vi "Begin.vi"(11 "Image Size":T4=enum."160x120") -> (0 "error out":errorcluster)   [LabVIEW 2012]
doc: "Called before other user functions, this VI is expected to open initial I/O refnums, load in file data, and do all program initialization. Notice that the <B>error out</B> terminal is simply used for data flow. Wiring it to other structures or subVIs ensures that this VI runs first."
uses:
  <vilib>/Rock Robotics/WPI/Camera/WPI_CameraImageSize.ctl
  <vilib>/Rock Robotics/SystemInterfaces/DIO/FPGA_DIOChannel.ctl
  <vilib>/Rock Robotics/WPI/Encoder/WPI_EncoderType.ctl
  <vilib>/Rock Robotics/SystemInterfaces/Typedef/FPGA_TypedefDigitalModule.ctl
  <vilib>/Rock Robotics/WPI/Camera/WPI_CameraWhite Balance Values.ctl
  <vilib>/Rock Robotics/WPI/Camera/WPI_CameraExposure Values.ctl
  <vilib>/Rock Robotics/WPI/Camera/WPI_CameraFrameRate.ctl
  <vilib>/Rock Robotics/WPI/DriverStation/WPI_DriverStationRobotMode2.ctl
  <vilib>/Rock Robotics/WPI/Joystick/WPI_JoystickDeviceEnum.ctl
  <vilib>/Rock Robotics/SystemInterfaces/Typedef/FPGA_TypedefAnalogModuleForGyro.ctl
  <vilib>/Rock Robotics/SystemInterfaces/AI/FPGA_AIGyroChannel.ctl
  <vilib>/Rock Robotics/WPI/SafetyOutput/WPI_SafetyOutputConfigMenu.ctl
  <vilib>/Rock Robotics/WPI/CAN/Jaguar/SubVIs/WPI_CANJaguar_ControlMode.ctl
  Robot Global Data.vi
  <vilib>/Rock Robotics/WPI/Counter/WPI_CounterDigitalInputToDigitalSource.vi
  <vilib>/Rock Robotics/WPI/MotorControl/WPI_MotorControlOpenCANJaguar.vi
  <vilib>/Rock Robotics/WPI/RobotDrive/WPI_RobotDriveOpen4MotorWithExistingMotors.vi
panel:
  in  "DIO Module":T1
  in  "Invert Direction":bool
  in  "Decoding Type":T2=enum."4x"
  in  "DistancePerCount (deg)":dbl=0.288
  in  "Encoder B Channel":T3=enum."DIO 2"
  in  "Encoder A Channel":T3
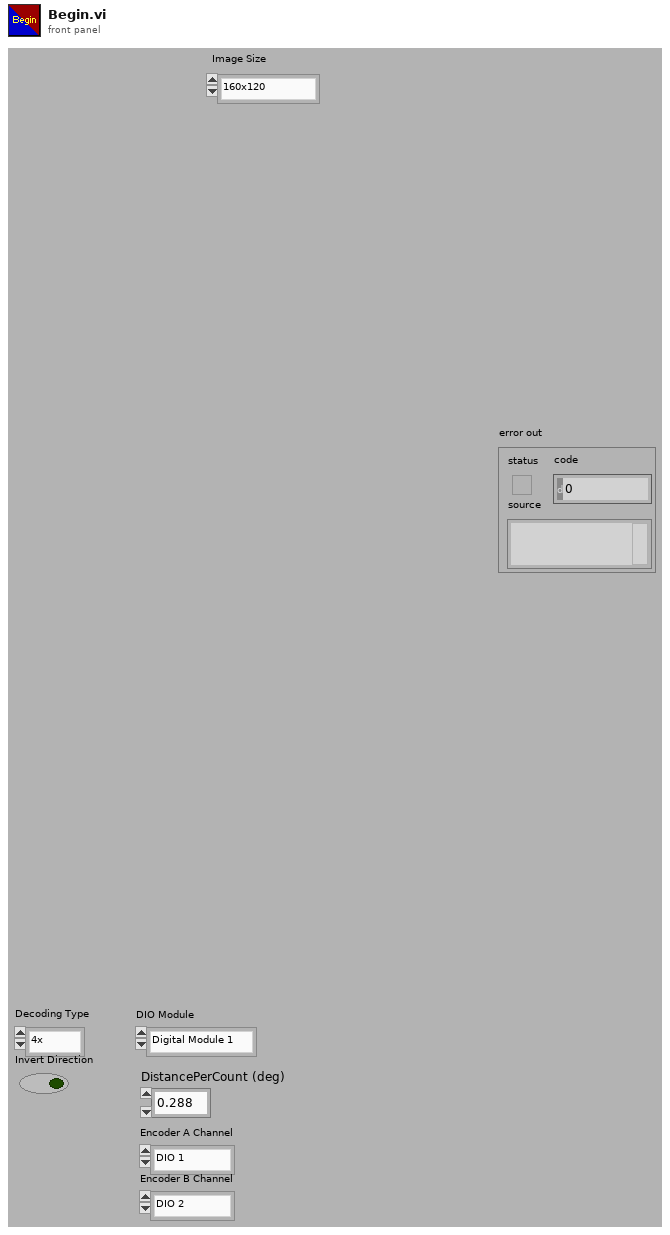
[diagram p1: front panel]
types:
  T1 = typedef "FPGA_TypedefDigitalModule.ctl" = enum16{"Digital Module 1", "Digital Module 2"}
  T2 = typedef "WPI_EncoderType.ctl" = enum16{"1x", "2x", "4x"}
  T3 = typedef "FPGA_DIOChannel.ctl" = enum8{"DIO 1", "DIO 2", "DIO 3", "DIO 4", "DIO 5", "DIO 6", "DIO 7", "DIO 8", "DIO 9", "DIO 10", "DIO 11", "DIO 12", "DIO 13", "DIO 14", "Invalid"}
  T4 = typedef "WPI_CameraImageSize.ctl" = enum16{"640x480", "320x240", "160x120"}
  T5 = typedef "WPI_CANJaguar_ControlMode.ctl" = enum8{"Percent VBus", "Current", "Speed", "Position", "Voltage"}
  T6 = typedef "WPI_SafetyOutputConfigMenu.ctl" = enum16{"Enable", "Disable"}
  T7 = typedef "FPGA_AIGyroChannel.ctl" = enum8{"AI 1", "AI 2", "Invalid"}
  T8 = typedef "FPGA_TypedefAnalogModuleForGyro.ctl" = enum16{"Analog Module 1"}
  T9 = typedef "WPI_JoystickDeviceEnum.ctl" = enum16{"USB 1", "USB 2", "USB 3", "USB 4", "Kinect 1", "Kinect 2"}
  T10 = typedef "WPI_DriverStationRobotMode2.ctl" = enum16{"Autonomous Disabled", "Autonomous Enabled", "Teleop Disabled", "Teleop Enabled", "Timeout", "Finish", "Test Disabled", "Test Enabled"}
  T11 = typedef "WPI_CameraFrameRate.ctl" = u32
  T12 = typedef "WPI_CameraExposure Values.ctl" = enum16{"Auto", "Flicker-free 50 Hz", "Flicker-free 60 Hz", "Hold current"}
  T13 = typedef "WPI_CameraWhite Balance Values.ctl" = enum16{"Auto", "Fixed indoor", "Fixed outdoor 1", "Fixed outdoor 2", "Fixed fluorescent 1", "Fixed fluorescent 2", "Hold current"}
  T14 = typedef "WPI_GyroDevRef.ctl" = cluster{"DevStatus":errorcluster, "Analog Module":T15, "Analog Channel":T16, "Offset":dbl, "Gain (VoltsPerDegree/Second)":dbl}
  T15 = typedef "FPGA_TypedefAnalogModule.ctl" = enum16{"Analog Module 1", "Analog Module 2"}
  T16 = typedef "FPGA_AIChannel.ctl" = enum8{"AI 1", "AI 2", "AI 3", "AI 4", "AI 5", "AI 6", "AI 7", "AI 8", "Invalid"}
  T17 = typedef "WPI_MotorControlDeviceRef.ctl" = cluster{"DeviceStatus":errorcluster, "Type":enum16{"PWM", "CAN"}, "PWM":cluster{"Digital Module":T1, "PWM Channel":T18, "DeadBand":T19}, "CAN":cluster{"Device Number":u8, "Control Mode":T5, "Semaphore":T20, "Max Vout":dbl}, "Invert":bool, "TransformRef":T21, "InvTransformRef":T21}
  T18 = typedef "FPGA_DIOPWMChannel.ctl" = enum8{"PWM 1", "PWM 2", "PWM 3", "PWM 4", "PWM 5", "PWM 6", "PWM 7", "PWM 8", "PWM 9", "PWM 10", "Invalid"}
  T19 = typedef "WPI_PWMDeadband.ctl" = cluster{"Name":string, "maxPositivePwm":i32, "minPositivePwm":i32, "centerPwm":i32, "maxNegativePwm":i32, "minNegativePwm":i32, "angularRange":u16}
  T20 = typedef "Semaphore RefNum" = refnum<k1>
  T21 = typedef "WPI_PWMTransform_ConPane.ctl" = refnum<vi>
  T22 = typedef "WPI_DigitalInputDevRef.ctl" = cluster{"DevStatus":errorcluster, "DIO Channel":T3, "Digital Module":T1}
  T23 = typedef "WPI_CameraDevRef.ctl" = cluster{"Camera Address":string, "CameraStatus":errorcluster, "Acquire Image Notifier":refnum<notifier>}
  T24 = typedef "WPI_JoystickDevRef.ctl" = cluster{"Device":T9}
  T25 = typedef "FPGA_CounterEncoderSourceConvertionLVSourceType.ctl" = cluster{"DevStatus":errorcluster, "AnalogTriggerMode?":bool, "DigitalMode":cluster{"Digital Module":T1, "DIO Channel":T26}, "AnalogTriggerMode":cluster{"AnalogTriggerIndex":T27, "OutputType":T28}}
  T26 = typedef "FPGA_DIODigitalSourceChannel.ctl" = enum8{"DIO 1", "DIO 2", "DIO 3", "DIO 4", "DIO 5", "DIO 6", "DIO 7", "DIO 8", "DIO 9", "DIO 10", "DIO 11", "DIO 12", "DIO 13", "DIO 14", "Disabled"}
  T27 = typedef "FPGA_AnalogTriggerIndex.ctl" = enum8{"Trig 0", "Trig 1", "Trig 2", "Trig 3", "Trig 4", "Trig 5", "Trig 6", "Trig 7", "Invalid"}
  T28 = typedef "FPGA_AnalogTriggerOutType.ctl" = enum16{"InWindow", "TriggerState", "Rising", "Falling"}
  T29 = typedef "WPI_EncoderDevRef.ctl" = cluster{"DevStatus":errorcluster, "EncoderIndex":T30, "CounterIndex":T31, "DistancePerCount":dbl, "Decoding Type":T2}
  T30 = typedef "FPGA_EncoderIdx.ctl" = enum8{"Enc 0", "Enc 1", "Enc 2", "Enc 3", "Invalid"}
  T31 = typedef "FPGA_CounterCtrSystemIndex.ctl" = enum8{"Ctr 0", "Ctr 1", "Ctr 2", "Ctr 3", "Ctr 4", "Ctr 5", "Ctr 6", "Ctr 7", "Invalid"}
  T32 = typedef "WPI_RobotDriveDevRef.ctl" = cluster{"DevStatus":errorcluster, "Motors[]":T17[], "Square Inputs":bool, "Max Output":dbl, "Isochronous":bool}
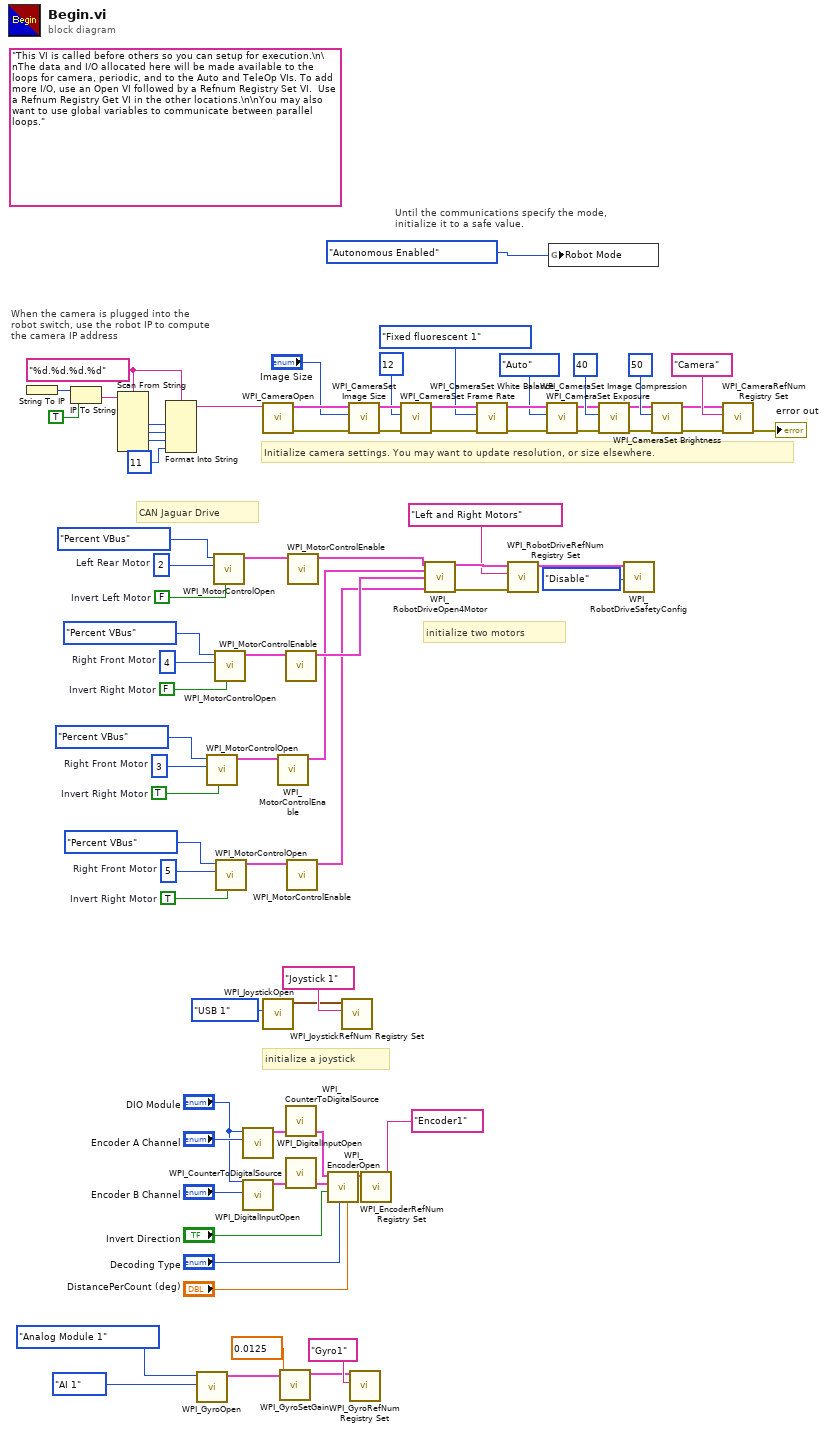
[diagram p0: block diagram]
diagram:
  w8 = TRUE  # Invert Right Motor
  w5 = 3  # Right Front Motor
  w12 = FALSE  # Invert Right Motor
  w9 = 4  # Right Front Motor
  w25 = FALSE  # Invert Left Motor
  w24 = TRUE  # Invert Right Motor
  w18 = 5  # Right Front Motor
  w20 = 2  # Left Rear Motor
  w50 = "%d.%d.%d.%d" ("format string")
  (unwired) "This VI is called before others so you can setup for execution.\n\nThe data and I/O allocated here will be made available to the loops for camera, periodic, and to the Auto and TeleOp VIs. To add more I/O, use an Open VI followed by a Refnum Registry Set VI.  Use a Refnum Registry Get VI in the other locations.\n\nYou may also want to use global variables to communicate between parallel loops."
  # "CAN Jaguar Drive"
  # "initialize two motors"
  # "initialize a joystick"
  # "Until the communications specify the mode,\ninitialize it to a safe value."
  # "When the camera is plugged into the\nrobot switch, use the robot IP to compute\nthe camera IP address"
  # "Initialize camera settings. You may want to update resolution, or size elsewhere."
  n1 = String To IP() -> (0:w57:u32)  [unwired: 1 in]
  n2 = IP To String(1:TRUE ("dot notation? (F)"), 2:w57) -> (0:w55:string)
  n3 = Scan From String(format string=w50, input string=w55) -> (output 1=w54:i32, output 2=w53:i32, output 3=w52:i32)  [unwired: 7 in, 3 out]
  n4 = Format Into String(format string=w50, w54, w53, w52, 11 ("Compression")) -> (resulting string=w48:string)  [unwired: 2 in, 1 out]
  n5 = call <vilib>:"WPI_GyroOpen.vi"("Analog Channel"=FPGA_AIGyroChannel."AI 1", "Analog Module (Module 1)"=FPGA_TypedefAnalogModuleForGyro."Analog Module 1") -> ("GyroDevRef"=w27:T14)  [unwired: 7 in, 2 out]
  n6 = call-poly <vilib>:"WPI_MotorControlOpen.vi"("Invert"=w8, "Device Number"=w5, "Control Mode"=WPI_CANJaguar_ControlMode."Percent VBus") -> ("MotorControlDeviceRef"=w7:T17)  [unwired: 3 in, 5 out]
  n7 = call-poly <vilib>:"WPI_MotorControlOpen.vi"("Invert"=w25, "Device Number"=w20, "Control Mode"=WPI_CANJaguar_ControlMode."Percent VBus") -> ("MotorControlDeviceRef"=w22:T17)  [unwired: 3 in, 5 out]
  n8 = call-poly <vilib>:"WPI_MotorControlOpen.vi"("Invert"=w12, "Device Number"=w9, "Control Mode"=WPI_CANJaguar_ControlMode."Percent VBus") -> ("MotorControlDeviceRef"=w11:T17)  [unwired: 3 in, 5 out]
  n9 = call-poly <vilib>:"WPI_MotorControlOpen.vi"("Invert"=w24, "Device Number"=w18, "Control Mode"=WPI_CANJaguar_ControlMode."Percent VBus") -> ("MotorControlDeviceRef"=w23:T17)  [unwired: 3 in, 5 out]
  n10 = call <vilib>:"WPI_DigitalInputOpen.vi"("DIO Channel"="Encoder A Channel", "Digital Module (Module 1)"="DIO Module") -> ("DigitalInputDevRef"=w41:T22)  [unwired: 1 in, 8 out]
  n11 = call <vilib>:"WPI_DigitalInputOpen.vi"("DIO Channel"="Encoder B Channel", "Digital Module (Module 1)"="DIO Module") -> ("DigitalInputDevRef"=w42:T22)  [unwired: 1 in, 8 out]
  n12 = call <vilib>:"WPI_CameraOpen.vi"("Camera Address"=w48) -> ("error out"=w69:errorcluster, "CameraDevRef"=w70:T23)  [unwired: 1 in, 8 out]
  n13 = call <vilib>:"WPI_JoystickOpen.vi"("JoystickDevice"=WPI_JoystickDeviceEnum."USB 1") -> ("JoystickDevRef"=w46:T24)  [unwired: 10 in]
  n14 = call <vilib>:"WPI_MotorControlEnable.vi"("CAN Jaguar Ref"=w7) -> ("CAN Jaguar Ref Out"=w2:T17)  [unwired: 9 in, 1 out]
  n15 = call <vilib>:"WPI_GyroSetGain.vi"("Gain (VoltsPerDegree/Second)"=0.0125, "GyroDevRef"=w27) -> ("GyroDevRef"=w26:T14)  [unwired: 8 in, 1 out]
  n16 = call <vilib>:"WPI_MotorControlEnable.vi"("CAN Jaguar Ref"=w11) -> ("CAN Jaguar Ref Out"=w3:T17)  [unwired: 9 in, 1 out]
  n17 = call-poly <vilib>:"WPI_CounterToDigitalSource.vi"("DigitalInputDevRef"=w41) -> ("Digital Source"=w40:T25)  [unwired: 6 out]
  n18 = call-poly <vilib>:"WPI_CounterToDigitalSource.vi"("DigitalInputDevRef"=w42) -> ("Digital Source"=w43:T25)  [unwired: 6 out]
  n19 = call <vilib>:"WPI_MotorControlEnable.vi"("CAN Jaguar Ref"=w23) -> ("CAN Jaguar Ref Out"=w1:T17)  [unwired: 9 in, 1 out]
  n20 = call <vilib>:"WPI_MotorControlEnable.vi"("CAN Jaguar Ref"=w22) -> ("CAN Jaguar Ref Out"=w4:T17)  [unwired: 9 in, 1 out]
  n21 = call <vilib>:"WPI_EncoderOpen.vi"("DistancePerCount"="DistancePerCount (deg)", "Decoding Type"="Decoding Type", "Invert Direction (False)"="Invert Direction", "BSource"=w43, "ASource"=w40) -> ("EncoderDevRef"=w34:T29)  [unwired: 3 in, 3 out]
  n22 = call <vilib>:"WPI_JoystickRefNum Registry Set.vi"("refnum name"="Joystick 1", "JoystickDevRef"=w46) -> ()  [unwired: 8 in, 2 out]
  n23 = call <vilib>:"WPI_CameraSet Image Size.vi"("error in (no error)"=w69, "Image Size"="Image Size", "CameraDevRef"=w70) -> ("error out"=w68:errorcluster, "CameraDevRef Out"=w71:T23)  [unwired: 7 out]
  n24 = call <vilib>:"WPI_GyroRefNum Registry Set.vi"("refnum name"="Gyro1", "GyroDevRef"=w26) -> ()  [unwired: 8 in, 2 out]
  n25 = call <vilib>:"WPI_EncoderRefNum Registry Set.vi"("refnum name"="Encoder1", "EncoderDevRef"=w34) -> ()  [unwired: 8 in, 2 out]
  n26 = call <vilib>:"WPI_CameraSet Frame Rate.vi"("error in (no error)"=w68, "Frame Rate (fps)"=T11 12, "CameraDevRef"=w71) -> ("error out"=w67:errorcluster, "CameraDevRef Out"=w73:T23)  [unwired: 7 out]
  n27 = call-poly <vilib>:"WPI_RobotDriveOpen4Motor.vi"("Rear Left Motor Dev Ref"=w4, "Rear Right Motor Dev Ref"=w2, "Front Left Motor Dev Ref"=w3, "Front Right Motor Dev Ref"=w1) -> ("RobotDriveDevRef"=w17:T32, "error out"=w15:errorcluster)  [unwired: 10 in]
  n28 = call <vilib>:"WPI_CameraSet White Balance.vi"("error in (no error)"=w67, "White Balance"=WPI_CameraWhite_Balance_Values."Fixed fluorescent 1", "CameraDevRef"=w73) -> ("error out"=w66:errorcluster, "CameraDevRef Out"=w72:T23)  [unwired: 7 out]
  n29 = call <vilib>:"WPI_RobotDriveRefNum Registry Set.vi"("error in (no error)"=w15, "refnum name"="Left and Right Motors", "RobotDriveDevRef"=w17) -> ("RobotDriveDevRef"=w14:T32)  [unwired: 8 out]
  n30 = call <vilib>:"WPI_CameraSet Exposure.vi"("error in (no error)"=w66, "Exposure"=WPI_CameraExposure_Values."Auto", "CameraDevRef"=w72) -> ("error out"=w65:errorcluster, "CameraDevRef Out"=w75:T23)  [unwired: 7 out]
  n31 = global write "Robot Global Data.vi" "Robot Mode"(WPI_DriverStationRobotMode2."Autonomous Enabled" ("Robot Mode")) -> ()
  n32 = call <vilib>:"WPI_CameraSet Image Compression.vi"("error in (no error)"=w65, "Compression"=40, "CameraDevRef"=w75) -> ("error out"=w64:errorcluster, "CameraDevRef Out"=w74:T23)  [unwired: 7 out]
  n33 = call <vilib>:"WPI_RobotDriveSafetyConfig.vi"("mode"=WPI_SafetyOutputConfigMenu."Disable", "RobotDriveDevRef"=w14) -> ()  [unwired: 8 in, 2 out]
  n34 = call <vilib>:"WPI_CameraSet Brightness.vi"("error in (no error)"=w64, "Brightness"=50, "CameraDevRef"=w74) -> ("error out"=w62:errorcluster, "CameraDevRef Out"=w63:T23)  [unwired: 7 out]
  n35 = call <vilib>:"WPI_CameraRefNum Registry Set.vi"("error in (no error)"=w62, "refnum name"="Camera", "CameraDevRef"=w63) -> ("error out"=→"error out":errorcluster)  [unwired: 8 out]
